vi "File2Array (SubVI).vi"(6 "Array for Processing":dbl[][](array[numeric]), 8 "error in (no error) in":errorcluster, 9 "File delimiter":string=",", 10 "Source array file":path, 11 "Load array from file?":bool) -> (0 "error in (no error) out":errorcluster, 3 "Loaded array":dbl[][](array[numeric]))   [LabVIEW 2016]
uses:
  <vilib>/Utility/file.llb/Read Delimited Spreadsheet (DBL).vi
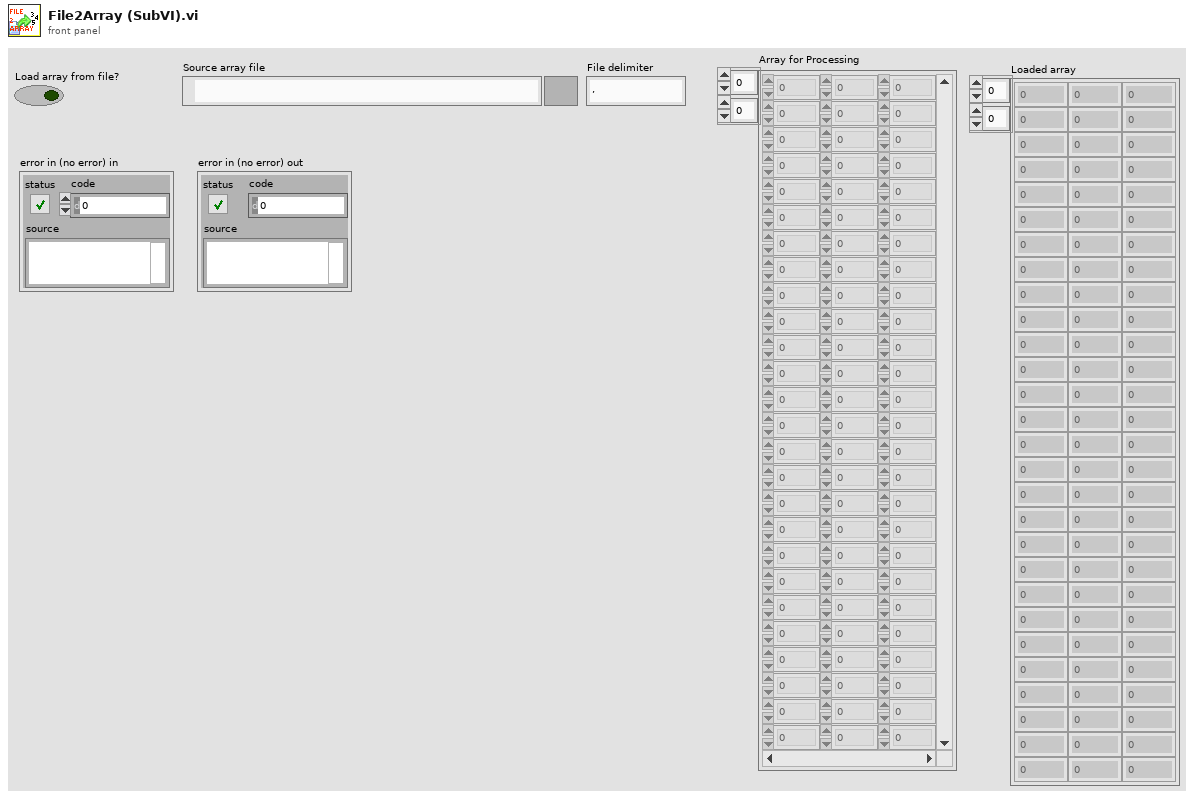
[diagram p1: front panel]
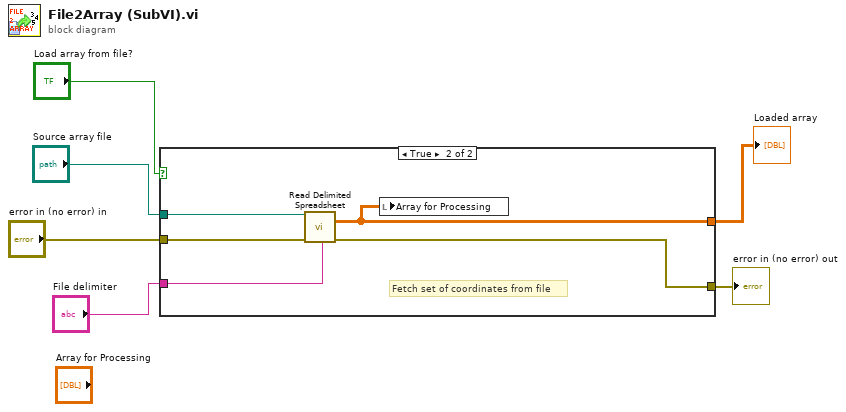
[diagram p0: block diagram]
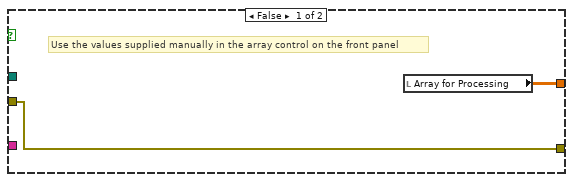
[diagram p2: hidden frame]
diagram:
  n1 = case shown="True" "Load array from file?" {
    tunnel: [w7 w10] -> w1
    tunnel: [w8 w9] -> w2
    tunnel: "error in (no error) in" -> [w8 w13]
    tunnel: "Source array file" -> [_ w12]
    tunnel: "File delimiter" -> [_ w11]
    frame False {
      # "Use the values supplied manually in the array control on the front panel"
      n2 = local read "Array for Processing"() -> (w7:dbl[][])
    }
    frame True {
      # "Fetch set of coordinates from file"
      n3 = call-poly <vilib>:"Read Delimited Spreadsheet.vi"("file path (dialog if empty)"=w12, "error in (no error)"=w13, "delimiter (\\t)"=w11) -> ("all rows"=w10:dbl[][], "error out"=w9:errorcluster)  [unwired: 7 in, 4 out]
      n4 = local write "Array for Processing"(w10) -> ()
    }
  }
  "error in (no error) out" <- w2
  "Loaded array" <- w1
